vi "uri parameter.vi"(8 "error in (no error)":errorcluster, 10 "zParam":string, 11 "zFilename":string) -> (0 "error out":errorcluster, 3 "function return":string)   [LabVIEW 2020, in "sqlite3.lvlib"]
uses:
  sqlite3.lvlib
  errstr.vi
  bin/sqlite3_64.dll
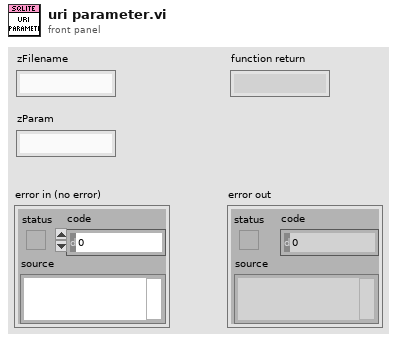
[diagram p1: front panel]
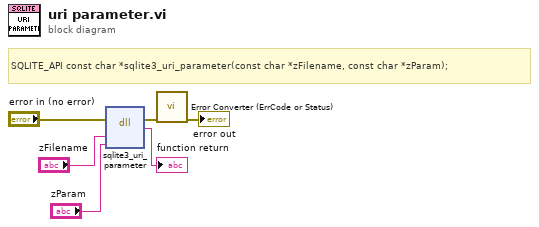
[diagram p0: block diagram]
diagram:
  # "SQLITE_API const char *sqlite3_uri_parameter(const char *zFilename, const char *zParam);"
  n1 = dll-call lib="D:/Project/Labview-Projects/database-configuration/externals/sqlite3/Source/bin/sqlite3_*.*" fn="sqlite3_uri_parameter"(error in="error in (no error)", "zFilename"="zFilename", "zParam"="zParam") -> (error out=w2:errorcluster, →"function return":string)  [unwired: 4 in, 1 out]
  n2 = call "Error Converter (ErrCode or Status).vi"("error in (no error)"=w2) -> ("error out"=→"error out":errorcluster)  [unwired: 10 in]
